vi "New Stuff.vi"(6 "Conditions":T2, 7 "Angular Accelerations":T3, 9 "Sample Period (s)":dbl, 10 "Limits":T1, 11 "Points in":cluster{"x":dbl, "y":dbl, "th":dbl}[](array[cluster])) -> (1 "result":bool)   [LabVIEW 2019]
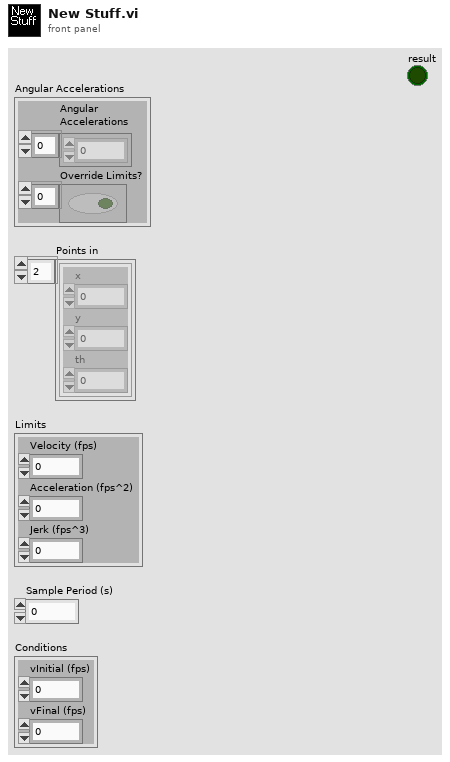
[diagram p1: front panel]
types:
  T1 = cluster{"Velocity (fps)":dbl, "Acceleration (fps^2)":dbl, "Jerk (fps^3)":dbl}
  T2 = cluster{"vInitial (fps)":dbl, "vFinal (fps)":dbl}
  T3 = cluster{"Angular \nAccelerations":dbl[], "Override Limits?":bool[]}
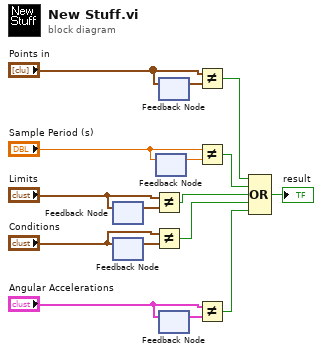
[diagram p0: block diagram]
diagram:
  n1 = feedback #1() -> (w11:T1)  [unwired: 1 in]
  n2 = feedback-in #1("Limits") -> ()
  n3 = feedback #2() -> (w13:T2)  [unwired: 1 in]
  n4 = feedback-in #2("Conditions") -> ()
  n5 = Not Equal?(x="Limits", y=w11) -> (x != y?=w3:bool)
  n6 = Not Equal?(x="Conditions", y=w13) -> (x != y?=w2:bool)
  n7 = feedback #3() -> (w7:dbl)  [unwired: 1 in]
  n8 = feedback-in #3("Sample Period (s)") -> ()
  n9 = feedback #4() -> (w9:cluster{"x":dbl, "y":dbl, "th":dbl}[])  [unwired: 1 in]
  n10 = feedback-in #4("Points in") -> ()
  n11 = feedback #5() -> (w15:T3)  [unwired: 1 in]
  n12 = feedback-in #5("Angular Accelerations") -> ()
  n13 = Not Equal?(x="Points in", y=w9) -> (x != y?=w4:bool)
  n14 = Not Equal?(x="Sample Period (s)", y=w7) -> (x != y?=w6:bool)
  n15 = Not Equal?(x="Angular Accelerations", y=w15) -> (x != y?=w1:bool)
  n16 = Compound Arithmetic op=OR(w4, w6, w3, w2, w1) -> (→"result":bool)
